vi "Build_History_Waveforms.vi"(9 "NoiseFloorSum":dbl, 10 "MaxValue Beac":dbl, 11 "MaxValue Cal":dbl) -> (2 "output cluster":T1)   [LabVIEW 2018]
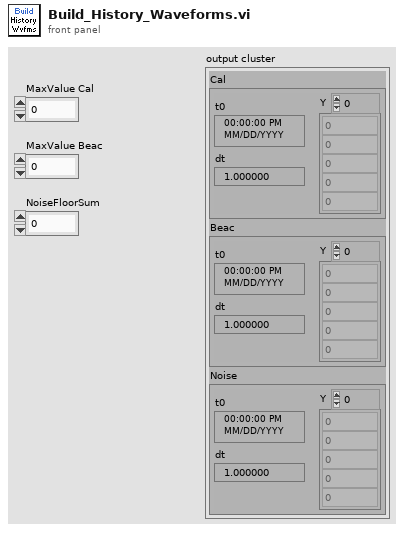
[diagram p1: front panel]
types:
  T1 = cluster{"Cal":waveform(dbl), "Beac":waveform(dbl), "Noise":waveform(dbl)}
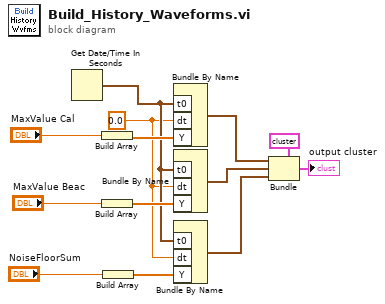
[diagram p0: block diagram]
diagram:
  w7 = 0.0 ("dt")
  n1 = Get Date/Time In Seconds() -> (seconds since 1Jan1904=w8:timestamp)
  n2 = Build Array("MaxValue Cal") -> (w10:dbl[])
  n3 = Build Array("MaxValue Beac") -> (w9:dbl[])
  n4 = Build Array("NoiseFloorSum") -> (w6:dbl[])
  n5 = Bundle By Name("t0"=w8, "dt"=w7, "Y"=w10) -> (w5:waveform(dbl))  [unwired: 1 in]
  n6 = Bundle By Name("t0"=w8, "dt"=w7, "Y"=w9) -> (w2:waveform(dbl))  [unwired: 1 in]
  n7 = Bundle By Name("t0"=w8, "dt"=w7, "Y"=w6) -> (w1:waveform(dbl))  [unwired: 1 in]
  n8 = Bundle(cluster=T1 {"Cal"={"t0"=timestamp(0 s since 1904-01-01), "dt"=1.0, "Y"=[]}, "Beac"={"t0"=timestamp(0 s since 1904-01-01), "dt"=1.0, "Y"=[]}, "Noise"={"t0"=timestamp(0 s since 1904-01-01), "dt"=1.0, "Y"=[]}}, "Cal"=w5, "Beac"=w2, "Noise"=w1) -> (→"output cluster":T1)
